vi "New Position.vi"(0 "Fruit in":refnum<class "Fruit.lvclass">, 5 "B Game Size":u16, 7 "Snake":refnum<class "Snake.lvclass">, 9 "Bomb":refnum<class "Bomb.lvclass">[](array[class]), 11 "error in (no error)":errorcluster) -> (4 "Fruit out":refnum<class "Fruit.lvclass">, 10 "Position":cluster{"X":dbl, "Y":dbl}, 15 "error out":errorcluster)   [LabVIEW 2021, in "Fruit.lvclass"]
uses:
  Fruit.lvclass
  C:/Users/poche/Programs/LabVIEW/imposible snake/GameEl_class/GameEl.lvclass
  Snake_class/Snake.lvclass
  Bomb/Bomb.lvclass
  GameEl_class/GameEl.lvclass/GameEl.ctl
  GameEl_class/Read position.vi
  GameEl_class/GameEl.lvclass
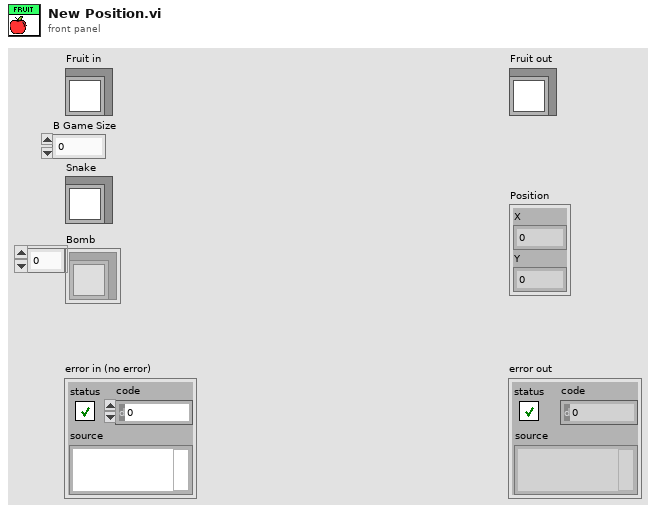
[diagram p1: front panel]
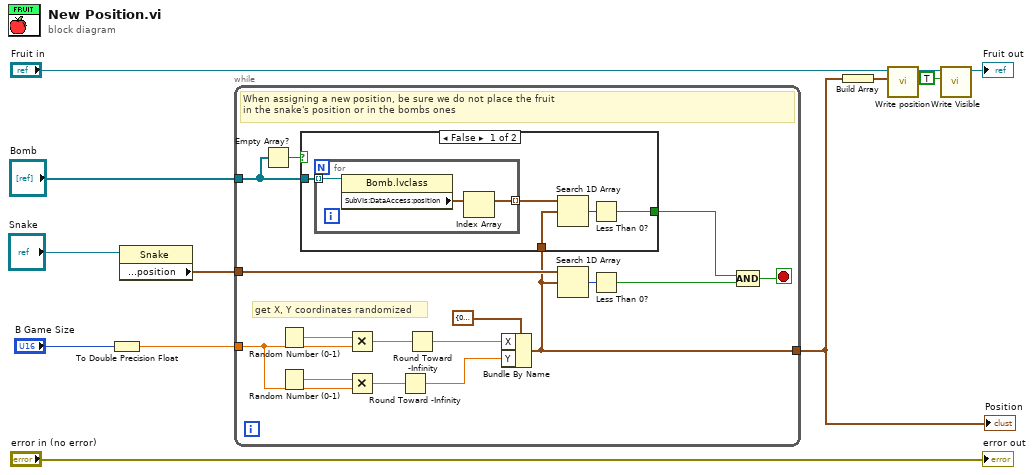
[diagram p0: block diagram]
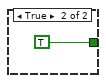
[diagram p2: hidden frame]
diagram:
  n1 = To Double Precision Float(number="B Game Size") -> (double precision float=w9:dbl)
  n2 = property class="Snake"(reference="Snake") -> ("SubVIs:DataAccess:position"=w7:cluster{"x":dbl, "y":dbl}[])  [unwired: 1 in, 2 out]
  n3 = while {
    tunnel: w9 -> [w26]
    tunnel: w7 -> [w19]
    tunnel: [w16] -> w4
    tunnel: "Bomb" -> [w14]
    stop <- w18 stop-if-true
    # "get X, Y coordinates randomized"
    # "When assigning a new position, be sure we do not place the fruit \nin the snake's position or in the bombs ones"
    n4 = Empty Array?(array=w14) -> (empty?=w13:bool)
    n5 = Random Number (0-1)() -> (number: 0 to 1=w28:dbl)
    n6 = Random Number (0-1)() -> (number: 0 to 1=w27:dbl)
    n7 = Multiply(x=w28, y=w26) -> (x*y=w24:dbl)
    n8 = Multiply(x=w27, y=w26) -> (x*y=w23:dbl)
    n9 = Round Toward -Infinity(1:w23) -> (0:w20:dbl)
    n10 = Round Toward -Infinity(1:w24) -> (0:w21:dbl)
    n11 = Bundle By Name(cluster=cluster{"X":dbl, "Y":dbl} {"X"=0.0, "Y"=0.0} ("Position"), "X"=w21, "Y"=w20) -> (w16:cluster{"X":dbl, "Y":dbl})
    n12 = case shown="False" w13 {
      tunnel: w16 -> [w32 _]
      tunnel: [w30 TRUE] -> w15
      tunnel: w14 -> [w29 _]
      frame False {
        n13 = for {
          tunnel: w29 -> [w36] mode=indexing
          tunnel: [w34] -> w33 mode=indexing
          n14 = property class="Bomb.lvclass"(reference=w36) -> ("SubVIs:DataAccess:position"=w35:cluster{"x":dbl, "y":dbl}[])  [unwired: 1 in, 2 out]
          n15 = Index Array(array=w35) -> (element=w34:cluster{"x":dbl, "y":dbl})  [unwired: 1 in]
        }
        n16 = Search 1D Array(1D array=w33, element=w32) -> (index of element=w31:i32)  [unwired: 1 in]
        n17 = Less Than 0?(x=w31) -> (x < 0?=w30:bool)
      }
      frame True {
      }
    }
    n18 = Search 1D Array(1D array=w19, element=w16) -> (index of element=w22:i32)  [unwired: 1 in]
    n19 = Less Than 0?(x=w22) -> (x < 0?=w17:bool)
    n20 = Compound Arithmetic op=AND(w15, w17) -> (w18:bool)
  }
  "Position" <- w4
  n21 = Build Array(w4) -> (w3:cluster{"X":dbl, "Y":dbl}[])
  n22 = call "Write position.vi"("position"=w3, "GameEl in"="Fruit in") -> ("GameEl out"=w5:refnum<class "Fruit.lvclass">)  [unwired: 8 in, 1 out]
  n23 = call "Write Visible.vi"("Visible"=TRUE, "GameEl in"=w5) -> ("GameEl out"=→"Fruit out":refnum<class "Fruit.lvclass">)  [unwired: 8 in, 1 out]
  "error out" <- "error in (no error)"
